vi "RTS MX4 Data.vi"(4 "Measurement Values in":dbl[][](array[numeric]), 6 "Debug":bool, 8 "Error In":errorcluster, 9 "Measurement Date Times":T1(array[cluster]), 10 "Chamber 1 Data in in":T4 {"Room PID Settings"."Room Dehumid Temperature I (*RM Dehum I1)" max=30000 step=1; "Room PID Settings"."Room Dehumid Temperature P (*RM Dehum P1)" max=30000 step=1; "Room PID Settings"."Room Cool Temperature I (*RM Cool I1)" max=30000 step=1; "Room PID Settings"."Room Cool Temperature P (*RM Cool P1)" max=30000 step=1; "Room PID Settings"."Room Heat I (*RM Heat I1)" max=30000 step=1; "Room PID Settings"."Room Heat P (*RM Heat P1)" max=30000 step=1; "Room PID Settings"."Room Humidity I (*RM Hum I1)" max=30000 step=1; "Room PID Settings"."Room Humidity P (*RM Hum P1)" max=30000 step=1; "Room PID Settings"."Room Dry I (*RM Dry I1)" max=30000 step=1; "Room PID Settings"."Room Dry P(*RM Dry P1)" max=30000 step=1; "Station 8"."Voltage (V):Element 1 Avg" format="%.3g"; "Station 8"."Voltage (V):Element 2 Avg" format="%.3g"; "Station 8"."Max Watt Hours" format="%.3g"; "Station 8"."Power Factor:Element 2" format="%.3g"; "Station 8"."Power Factor:Element 1" format="%.3g"; "Station 8"."Apparent Power (VA):Element 2" format="%.3g"; "Station 8"."Apparent Power (VA):Element 1" format="%.3g"; "Station 8"."Frequency (Hz):Element 1" format="%.3g"; "Station 8"."Time:Element 1" format="%.3g"; "Station 8"."Voltage Crest Factor:Element 2" format="%.3g"; "Station 8"."Voltage Crest Factor:Element 1" format="%.3g"; "Station 8"."Voltage Harmonic (%):Element 2" format="%.3g"; "Station 8"."Voltage Harmonic (%):Element 1" format="%.3g"; "Station 8"."Current Crest Factor:Element 2" format="%.3g"; "Station 8"."Current Crest Factor:Element 1" format="%.3g"; "Station 8"."Voltage (V):Element 1" format="%.3g"; "Station 8"."Voltage (V):Element 2" format="%.3g"; "Station 8"."Watt Hours (Wh):Sigma" format="%.3f"; "Station 8"."Power (W):Sigma" format="%.3g"; "Station 8"."Current (A):Element 2" format="%.3g"; "Station 8"."Current (A):Element 1" format="%.3g"; "Station 7"."Voltage (V):Element 1 Avg" format="%.3g"; "Station 7"."Voltage (V):Element 2 Avg" format="%.3g"; "Station 7"."Max Watt Hours" format="%.3g"; "Station 7"."Power Factor:Element 2" format="%.3g"; "Station 7"."Power Factor:Element 1" format="%.3g"; "Station 7"."Apparent Power (VA):Element 2" format="%.3g"; "Station 7"."Apparent Power (VA):Element 1" format="%.3g"; "Station 7"."Frequency (Hz):Element 1" format="%.3g"; "Station 7"."Time:Element 1" format="%.3g"; "Station 7"."Voltage Crest Factor:Element 2" format="%.3g"; "Station 7"."Voltage Crest Factor:Element 1" format="%.3g"; "Station 7"."Voltage Harmonic (%):Element 2" format="%.3g"; "Station 7"."Voltage Harmonic (%):Element 1" format="%.3g"; "Station 7"."Current Crest Factor:Element 2" format="%.3g"; "Station 7"."Current Crest Factor:Element 1" format="%.3g"; "Station 7"."Voltage (V):Element 1" format="%.3g"; "Station 7"."Voltage (V):Element 2" format="%.3g"; "Station 7"."Watt Hours (Wh):Sigma" format="%.3f"; "Station 7"."Power (W):Sigma" format="%.3g"; "Station 7"."Current (A):Element 2" format="%.3g"; "Station 7"."Current (A):Element 1" format="%.3g"; "Station 6"."Voltage (V):Element 1 Avg" format="%.3g"; "Station 6"."Voltage (V):Element 2 Avg" format="%.3g"; "Station 6"."Max Watt Hours" format="%.3g"; "Station 6"."Power Factor:Element 2" format="%.3g"; "Station 6"."Power Factor:Element 1" format="%.3g"; "Station 6"."Apparent Power (VA):Element 2" format="%.3g"; "Station 6"."Apparent Power (VA):Element 1" format="%.3g"; "Station 6"."Frequency (Hz):Element 1" format="%.3g"; "Station 6"."Time:Element 1" format="%.3g"; "Station 6"."Voltage Crest Factor:Element 2" format="%.3g"; "Station 6"."Voltage Crest Factor:Element 1" format="%.3g"; "Station 6"."Voltage Harmonic (%):Element 2" format="%.3g"; "Station 6"."Voltage Harmonic (%):Element 1" format="%.3g"; "Station 6"."Current Crest Factor:Element 2" format="%.3g"; "Station 6"."Current Crest Factor:Element 1" format="%.3g"; "Station 6"."Voltage (V):Element 1" format="%.3g"; "Station 6"."Voltage (V):Element 2" format="%.3g"; "Station 6"."Watt Hours (Wh):Sigma" format="%.3f"; "Station 6"."Power (W):Sigma" format="%.3g"; "Station 6"."Current (A):Element 2" format="%.3g"; "Station 6"."Current (A):Element 1" format="%.3g"; "Station 5"."Voltage (V):Element 1 Avg" format="%.3g"; "Station 5"."Voltage (V):Element 2 Avg" format="%.3g"; "Station 5"."Max Watt Hours" format="%.3g"; "Station 5"."Power Factor:Element 2" format="%.3g"; "Station 5"."Power Factor:Element 1" format="%.3g"; "Station 5"."Apparent Power (VA):Element 2" format="%.3g"; "Station 5"."Apparent Power (VA):Element 1" format="%.3g"; "Station 5"."Frequency (Hz):Element 1" format="%.3g"; "Station 5"."Time:Element 1" format="%.3g"; "Station 5"."Voltage Crest Factor:Element 2" format="%.3g"; "Station 5"."Voltage Crest Factor:Element 1" format="%.3g"; "Station 5"."Voltage Harmonic (%):Element 2" format="%.3g"; "Station 5"."Voltage Harmonic (%):Element 1" format="%.3g"; "Station 5"."Current Crest Factor:Element 2" format="%.3g"; "Station 5"."Current Crest Factor:Element 1" format="%.3g"; "Station 5"."Voltage (V):Element 1" format="%.3g"; "Station 5"."Voltage (V):Element 2" format="%.3g"; "Station 5"."Watt Hours (Wh):Sigma" format="%.3f"; "Station 5"."Power (W):Sigma" format="%.3g"; "Station 5"."Current (A):Element 2" format="%.3g"; "Station 5"."Current (A):Element 1" format="%.3g"; "Station 4"."Voltage (V):Element 1 Avg" format="%.3g"; "Station 4"."Voltage (V):Element 2 Avg" format="%.3g"; "Station 4"."Max Watt Hours" format="%.3g"; "Station 4"."Power Factor:Element 2" format="%.3g"; "Station 4"."Power Factor:Element 1" format="%.3g"; "Station 4"."Apparent Power (VA):Element 2" format="%.3g"; "Station 4"."Apparent Power (VA):Element 1" format="%.3g"; "Station 4"."Frequency (Hz):Element 1" format="%.3g"; "Station 4"."Time:Element 1" format="%.3g"; "Station 4"."Voltage Crest Factor:Element 2" format="%.3g"; "Station 4"."Voltage Crest Factor:Element 1" format="%.3g"; "Station 4"."Voltage Harmonic (%):Element 2" format="%.3g"; "Station 4"."Voltage Harmonic (%):Element 1" format="%.3g"; "Station 4"."Current Crest Factor:Element 2" format="%.3g"; "Station 4"."Current Crest Factor:Element 1" format="%.3g"; "Station 4"."Voltage (V):Element 1" format="%.3g"; "Station 4"."Voltage (V):Element 2" format="%.3g"; "Station 4"."Watt Hours (Wh):Sigma" format="%.3f"; "Station 4"."Power (W):Sigma" format="%.3g"; "Station 4"."Current (A):Element 2" format="%.3g"; "Station 4"."Current (A):Element 1" format="%.3g"; "Station 3"."Voltage (V):Element 1 Avg" format="%.3g"; "Station 3"."Voltage (V):Element 2 Avg" format="%.3g"; "Station 3"."Max Watt Hours" format="%.3g"; "Station 3"."Power Factor:Element 2" format="%.3g"; "Station 3"."Power Factor:Element 1" format="%.3g"; "Station 3"."Apparent Power (VA):Element 2" format="%.3g"; "Station 3"."Apparent Power (VA):Element 1" format="%.3g"; "Station 3"."Frequency (Hz):Element 1" format="%.3g"; "Station 3"."Time:Element 1" format="%.3g"; "Station 3"."Voltage Crest Factor:Element 2" format="%.3g"; "Station 3"."Voltage Crest Factor:Element 1" format="%.3g"; "Station 3"."Voltage Harmonic (%):Element 2" format="%.3g"; "Station 3"."Voltage Harmonic (%):Element 1" format="%.3g"; "Station 3"."Current Crest Factor:Element 2" format="%.3g"; "Station 3"."Current Crest Factor:Element 1" format="%.3g"; "Station 3"."Voltage (V):Element 1" format="%.3g"; "Station 3"."Voltage (V):Element 2" format="%.3g"; "Station 3"."Watt Hours (Wh):Sigma" format="%.3f"; "Station 3"."Power (W):Sigma" format="%.3g"; "Station 3"."Current (A):Element 2" format="%.3g"; "Station 3"."Current (A):Element 1" format="%.3g"; "Station 2"."Voltage (V):Element 1 Avg" format="%.3g"; "Station 2"."Voltage (V):Element 2 Avg" format="%.3g"; "Station 2"."Max Watt Hours" format="%.3g"; "Station 2"."Power Factor:Element 2" format="%.3g"; "Station 2"."Power Factor:Element 1" format="%.3g"; "Station 2"."Apparent Power (VA):Element 2" format="%.3g"; "Station 2"."Apparent Power (VA):Element 1" format="%.3g"; "Station 2"."Frequency (Hz):Element 1" format="%.3g"; "Station 2"."Time:Element 1" format="%.3g"; "Station 2"."Voltage Crest Factor:Element 2" format="%.3g"; "Station 2"."Voltage Crest Factor:Element 1" format="%.3g"; "Station 2"."Voltage Harmonic (%):Element 2" format="%.3g"; "Station 2"."Voltage Harmonic (%):Element 1" format="%.3g"; "Station 2"."Current Crest Factor:Element 2" format="%.3g"; "Station 2"."Current Crest Factor:Element 1" format="%.3g"; "Station 2"."Voltage (V):Element 1" format="%.3g"; "Station 2"."Voltage (V):Element 2" format="%.3g"; "Station 2"."Watt Hours (Wh):Sigma" format="%.3f"; "Station 2"."Power (W):Sigma" format="%.3g"; "Station 2"."Current (A):Element 2" format="%.3g"; "Station 2"."Current (A):Element 1" format="%.3g"; "Station 1"."Voltage (V):Element 1 Avg" format="%.3g"; "Station 1"."Voltage (V):Element 2 Avg" format="%.3g"; "Station 1"."Max Watt Hours" format="%.3g"; "Station 1"."Power Factor:Element 2" format="%.3g"; "Station 1"."Power Factor:Element 1" format="%.3g"; "Station 1"."Apparent Power (VA):Element 2" format="%.3g"; "Station 1"."Apparent Power (VA):Element 1" format="%.3g"; "Station 1"."Frequency (Hz):Element 1" format="%.3g"; "Station 1"."Time:Element 1" format="%.3g"; "Station 1"."Voltage Crest Factor:Element 2" format="%.3g"; "Station 1"."Voltage Crest Factor:Element 1" format="%.3g"; "Station 1"."Voltage Harmonic (%):Element 2" format="%.3g"; "Station 1"."Voltage Harmonic (%):Element 1" format="%.3g"; "Station 1"."Current Crest Factor:Element 2" format="%.3g"; "Station 1"."Current Crest Factor:Element 1" format="%.3g"; "Station 1"."Voltage (V):Element 1" format="%.3g"; "Station 1"."Voltage (V):Element 2" format="%.3g"; "Station 1"."Watt Hours (Wh):Sigma" format="%.3f"; "Station 1"."Power (W):Sigma" format="%.3g"; "Station 1"."Current (A):Element 2" format="%.3g"; "Station 1"."Current (A):Element 1" format="%.3g"}, 11 "MX":T2={"Base Time"=0, "Session Number"=0, "Last Data Number"={"High"=-1, "Low"=4294967295}, "Channel List"=[], "FIFO Number (0)"=0, "Channel Number (1)"=1, "Select FIFO or Channel (F:Channel)"=FALSE, "MX100 Data"={"Measurement Values out"=[], "Date/Time"=""}} {"Channel Number (1)" min=1 max=60 step=1; "FIFO Number (0)" min=-1 max=2 step=1}) -> (0 "Error Out":errorcluster, 2 "Chamber 1 Data out":T4 {"Room PID Settings"."Room Dehumid Temperature I (*RM Dehum I1)" max=30000 step=1; "Room PID Settings"."Room Dehumid Temperature P (*RM Dehum P1)" max=30000 step=1; "Room PID Settings"."Room Cool Temperature I (*RM Cool I1)" max=30000 step=1; "Room PID Settings"."Room Cool Temperature P (*RM Cool P1)" max=30000 step=1; "Room PID Settings"."Room Heat I (*RM Heat I1)" max=30000 step=1; "Room PID Settings"."Room Heat P (*RM Heat P1)" max=30000 step=1; "Room PID Settings"."Room Humidity I (*RM Hum I1)" max=30000 step=1; "Room PID Settings"."Room Humidity P (*RM Hum P1)" max=30000 step=1; "Room PID Settings"."Room Dry I (*RM Dry I1)" max=30000 step=1; "Room PID Settings"."Room Dry P(*RM Dry P1)" max=30000 step=1; "Station 8"."Voltage (V):Element 1 Avg" format="%.3g"; "Station 8"."Voltage (V):Element 2 Avg" format="%.3g"; "Station 8"."Max Watt Hours" format="%.3g"; "Station 8"."Power Factor:Element 2" format="%.3g"; "Station 8"."Power Factor:Element 1" format="%.3g"; "Station 8"."Apparent Power (VA):Element 2" format="%.3g"; "Station 8"."Apparent Power (VA):Element 1" format="%.3g"; "Station 8"."Frequency (Hz):Element 1" format="%.3g"; "Station 8"."Time:Element 1" format="%.3g"; "Station 8"."Voltage Crest Factor:Element 2" format="%.3g"; "Station 8"."Voltage Crest Factor:Element 1" format="%.3g"; "Station 8"."Voltage Harmonic (%):Element 2" format="%.3g"; "Station 8"."Voltage Harmonic (%):Element 1" format="%.3g"; "Station 8"."Current Crest Factor:Element 2" format="%.3g"; "Station 8"."Current Crest Factor:Element 1" format="%.3g"; "Station 8"."Voltage (V):Element 1" format="%.3g"; "Station 8"."Voltage (V):Element 2" format="%.3g"; "Station 8"."Watt Hours (Wh):Sigma" format="%.3f"; "Station 8"."Power (W):Sigma" format="%.3g"; "Station 8"."Current (A):Element 2" format="%.3g"; "Station 8"."Current (A):Element 1" format="%.3g"; "Station 7"."Voltage (V):Element 1 Avg" format="%.3g"; "Station 7"."Voltage (V):Element 2 Avg" format="%.3g"; "Station 7"."Max Watt Hours" format="%.3g"; "Station 7"."Power Factor:Element 2" format="%.3g"; "Station 7"."Power Factor:Element 1" format="%.3g"; "Station 7"."Apparent Power (VA):Element 2" format="%.3g"; "Station 7"."Apparent Power (VA):Element 1" format="%.3g"; "Station 7"."Frequency (Hz):Element 1" format="%.3g"; "Station 7"."Time:Element 1" format="%.3g"; "Station 7"."Voltage Crest Factor:Element 2" format="%.3g"; "Station 7"."Voltage Crest Factor:Element 1" format="%.3g"; "Station 7"."Voltage Harmonic (%):Element 2" format="%.3g"; "Station 7"."Voltage Harmonic (%):Element 1" format="%.3g"; "Station 7"."Current Crest Factor:Element 2" format="%.3g"; "Station 7"."Current Crest Factor:Element 1" format="%.3g"; "Station 7"."Voltage (V):Element 1" format="%.3g"; "Station 7"."Voltage (V):Element 2" format="%.3g"; "Station 7"."Watt Hours (Wh):Sigma" format="%.3f"; "Station 7"."Power (W):Sigma" format="%.3g"; "Station 7"."Current (A):Element 2" format="%.3g"; "Station 7"."Current (A):Element 1" format="%.3g"; "Station 6"."Voltage (V):Element 1 Avg" format="%.3g"; "Station 6"."Voltage (V):Element 2 Avg" format="%.3g"; "Station 6"."Max Watt Hours" format="%.3g"; "Station 6"."Power Factor:Element 2" format="%.3g"; "Station 6"."Power Factor:Element 1" format="%.3g"; "Station 6"."Apparent Power (VA):Element 2" format="%.3g"; "Station 6"."Apparent Power (VA):Element 1" format="%.3g"; "Station 6"."Frequency (Hz):Element 1" format="%.3g"; "Station 6"."Time:Element 1" format="%.3g"; "Station 6"."Voltage Crest Factor:Element 2" format="%.3g"; "Station 6"."Voltage Crest Factor:Element 1" format="%.3g"; "Station 6"."Voltage Harmonic (%):Element 2" format="%.3g"; "Station 6"."Voltage Harmonic (%):Element 1" format="%.3g"; "Station 6"."Current Crest Factor:Element 2" format="%.3g"; "Station 6"."Current Crest Factor:Element 1" format="%.3g"; "Station 6"."Voltage (V):Element 1" format="%.3g"; "Station 6"."Voltage (V):Element 2" format="%.3g"; "Station 6"."Watt Hours (Wh):Sigma" format="%.3f"; "Station 6"."Power (W):Sigma" format="%.3g"; "Station 6"."Current (A):Element 2" format="%.3g"; "Station 6"."Current (A):Element 1" format="%.3g"; "Station 5"."Voltage (V):Element 1 Avg" format="%.3g"; "Station 5"."Voltage (V):Element 2 Avg" format="%.3g"; "Station 5"."Max Watt Hours" format="%.3g"; "Station 5"."Power Factor:Element 2" format="%.3g"; "Station 5"."Power Factor:Element 1" format="%.3g"; "Station 5"."Apparent Power (VA):Element 2" format="%.3g"; "Station 5"."Apparent Power (VA):Element 1" format="%.3g"; "Station 5"."Frequency (Hz):Element 1" format="%.3g"; "Station 5"."Time:Element 1" format="%.3g"; "Station 5"."Voltage Crest Factor:Element 2" format="%.3g"; "Station 5"."Voltage Crest Factor:Element 1" format="%.3g"; "Station 5"."Voltage Harmonic (%):Element 2" format="%.3g"; "Station 5"."Voltage Harmonic (%):Element 1" format="%.3g"; "Station 5"."Current Crest Factor:Element 2" format="%.3g"; "Station 5"."Current Crest Factor:Element 1" format="%.3g"; "Station 5"."Voltage (V):Element 1" format="%.3g"; "Station 5"."Voltage (V):Element 2" format="%.3g"; "Station 5"."Watt Hours (Wh):Sigma" format="%.3f"; "Station 5"."Power (W):Sigma" format="%.3g"; "Station 5"."Current (A):Element 2" format="%.3g"; "Station 5"."Current (A):Element 1" format="%.3g"; "Station 4"."Voltage (V):Element 1 Avg" format="%.3g"; "Station 4"."Voltage (V):Element 2 Avg" format="%.3g"; "Station 4"."Max Watt Hours" format="%.3g"; "Station 4"."Power Factor:Element 2" format="%.3g"; "Station 4"."Power Factor:Element 1" format="%.3g"; "Station 4"."Apparent Power (VA):Element 2" format="%.3g"; "Station 4"."Apparent Power (VA):Element 1" format="%.3g"; "Station 4"."Frequency (Hz):Element 1" format="%.3g"; "Station 4"."Time:Element 1" format="%.3g"; "Station 4"."Voltage Crest Factor:Element 2" format="%.3g"; "Station 4"."Voltage Crest Factor:Element 1" format="%.3g"; "Station 4"."Voltage Harmonic (%):Element 2" format="%.3g"; "Station 4"."Voltage Harmonic (%):Element 1" format="%.3g"; "Station 4"."Current Crest Factor:Element 2" format="%.3g"; "Station 4"."Current Crest Factor:Element 1" format="%.3g"; "Station 4"."Voltage (V):Element 1" format="%.3g"; "Station 4"."Voltage (V):Element 2" format="%.3g"; "Station 4"."Watt Hours (Wh):Sigma" format="%.3f"; "Station 4"."Power (W):Sigma" format="%.3g"; "Station 4"."Current (A):Element 2" format="%.3g"; "Station 4"."Current (A):Element 1" format="%.3g"; "Station 3"."Voltage (V):Element 1 Avg" format="%.3g"; "Station 3"."Voltage (V):Element 2 Avg" format="%.3g"; "Station 3"."Max Watt Hours" format="%.3g"; "Station 3"."Power Factor:Element 2" format="%.3g"; "Station 3"."Power Factor:Element 1" format="%.3g"; "Station 3"."Apparent Power (VA):Element 2" format="%.3g"; "Station 3"."Apparent Power (VA):Element 1" format="%.3g"; "Station 3"."Frequency (Hz):Element 1" format="%.3g"; "Station 3"."Time:Element 1" format="%.3g"; "Station 3"."Voltage Crest Factor:Element 2" format="%.3g"; "Station 3"."Voltage Crest Factor:Element 1" format="%.3g"; "Station 3"."Voltage Harmonic (%):Element 2" format="%.3g"; "Station 3"."Voltage Harmonic (%):Element 1" format="%.3g"; "Station 3"."Current Crest Factor:Element 2" format="%.3g"; "Station 3"."Current Crest Factor:Element 1" format="%.3g"; "Station 3"."Voltage (V):Element 1" format="%.3g"; "Station 3"."Voltage (V):Element 2" format="%.3g"; "Station 3"."Watt Hours (Wh):Sigma" format="%.3f"; "Station 3"."Power (W):Sigma" format="%.3g"; "Station 3"."Current (A):Element 2" format="%.3g"; "Station 3"."Current (A):Element 1" format="%.3g"; "Station 2"."Voltage (V):Element 1 Avg" format="%.3g"; "Station 2"."Voltage (V):Element 2 Avg" format="%.3g"; "Station 2"."Max Watt Hours" format="%.3g"; "Station 2"."Power Factor:Element 2" format="%.3g"; "Station 2"."Power Factor:Element 1" format="%.3g"; "Station 2"."Apparent Power (VA):Element 2" format="%.3g"; "Station 2"."Apparent Power (VA):Element 1" format="%.3g"; "Station 2"."Frequency (Hz):Element 1" format="%.3g"; "Station 2"."Time:Element 1" format="%.3g"; "Station 2"."Voltage Crest Factor:Element 2" format="%.3g"; "Station 2"."Voltage Crest Factor:Element 1" format="%.3g"; "Station 2"."Voltage Harmonic (%):Element 2" format="%.3g"; "Station 2"."Voltage Harmonic (%):Element 1" format="%.3g"; "Station 2"."Current Crest Factor:Element 2" format="%.3g"; "Station 2"."Current Crest Factor:Element 1" format="%.3g"; "Station 2"."Voltage (V):Element 1" format="%.3g"; "Station 2"."Voltage (V):Element 2" format="%.3g"; "Station 2"."Watt Hours (Wh):Sigma" format="%.3f"; "Station 2"."Power (W):Sigma" format="%.3g"; "Station 2"."Current (A):Element 2" format="%.3g"; "Station 2"."Current (A):Element 1" format="%.3g"; "Station 1"."Voltage (V):Element 1 Avg" format="%.3g"; "Station 1"."Voltage (V):Element 2 Avg" format="%.3g"; "Station 1"."Max Watt Hours" format="%.3g"; "Station 1"."Power Factor:Element 2" format="%.3g"; "Station 1"."Power Factor:Element 1" format="%.3g"; "Station 1"."Apparent Power (VA):Element 2" format="%.3g"; "Station 1"."Apparent Power (VA):Element 1" format="%.3g"; "Station 1"."Frequency (Hz):Element 1" format="%.3g"; "Station 1"."Time:Element 1" format="%.3g"; "Station 1"."Voltage Crest Factor:Element 2" format="%.3g"; "Station 1"."Voltage Crest Factor:Element 1" format="%.3g"; "Station 1"."Voltage Harmonic (%):Element 2" format="%.3g"; "Station 1"."Voltage Harmonic (%):Element 1" format="%.3g"; "Station 1"."Current Crest Factor:Element 2" format="%.3g"; "Station 1"."Current Crest Factor:Element 1" format="%.3g"; "Station 1"."Voltage (V):Element 1" format="%.3g"; "Station 1"."Voltage (V):Element 2" format="%.3g"; "Station 1"."Watt Hours (Wh):Sigma" format="%.3f"; "Station 1"."Power (W):Sigma" format="%.3g"; "Station 1"."Current (A):Element 2" format="%.3g"; "Station 1"."Current (A):Element 1" format="%.3g"})   [LabVIEW 2016]
uses:
  Type Definitions/RTS Chamber Data.ctl
  Utility/Type Definitions/UTILITY Power Data.ctl
  Type Definitions/RTS Chamber TCs.ctl
  Type Definitions/RTS MX5 AUX Data.ctl
  Drivers/WAGO 750-881/Type Definitions/Wago Door Relays.ctl
  Drivers/WAGO 750-881/Type Definitions/Wago Contactor Settings.ctl
  Drivers/WAGO 750-881/Type Definitions/Wago Ground Leakage.ctl
  Drivers/WAGO 750-881/Type Definitions/Wago Measured Input Data.ctl
  Drivers/WAGO 750-881/Type Definitions/Wago Room Setpoint Targets.ctl
  Drivers/WAGO 750-881/Type Definitions/Wago Room PID Settings.ctl
  Drivers/WAGO 750-881/Type Definitions/Wago Room Condtions.ctl
  Drivers/Yokogawa MX100/Type Definitions/MX100 Initialization.ctl
  Drivers/Yokogawa MX100/Type Definitions/MX100 Data.ctl
panel:
  # "APLUS"
  # "MX100"
  # "Wago Controller"
  # "APLUS"
  # "MX100"
  # "Wago Controller"
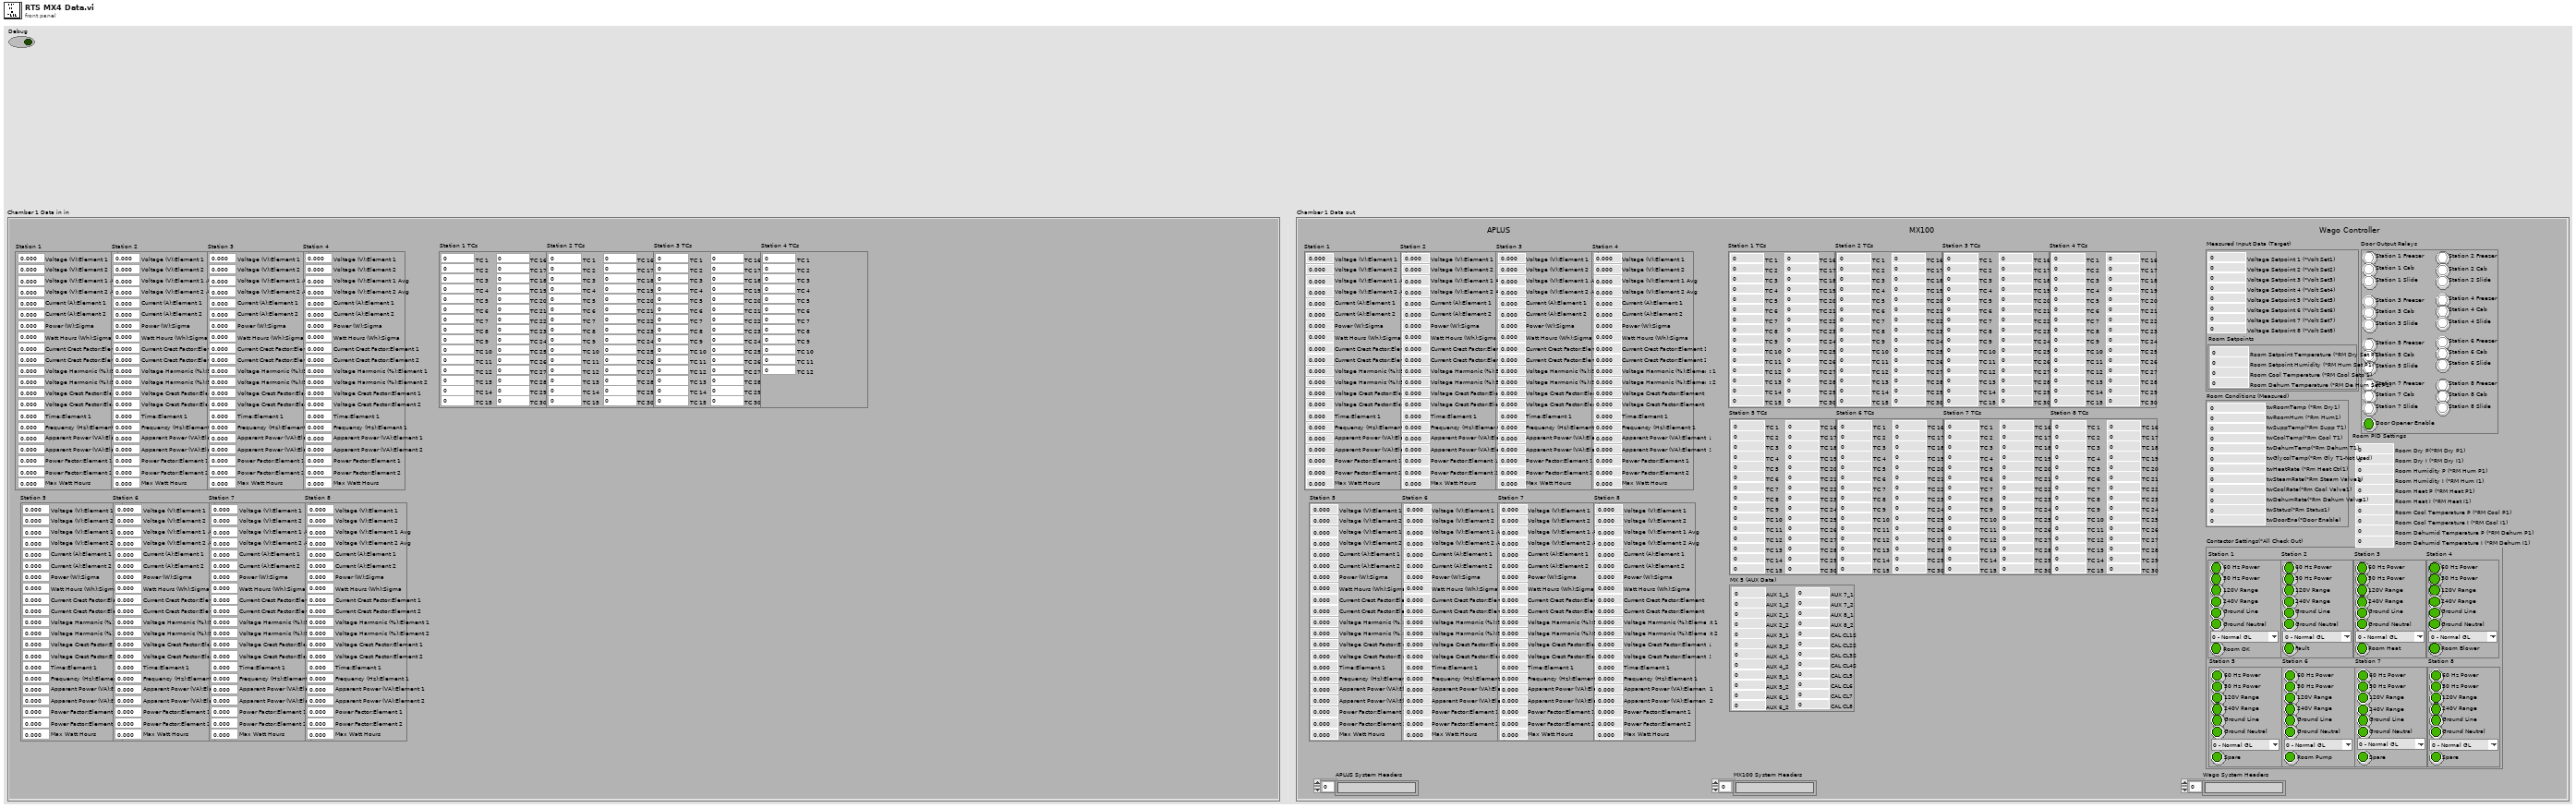
[diagram p1: front panel]
types:
  T1 = cluster{"Measurement Time":u32, "Milli Second":i32}[]
  T2 = typedef "MX100 Initialization.ctl" = cluster{"Base Time":i32, "Session Number":i32, "Last Data Number":cluster{"High":i32, "Low":u32}, "Channel List":string[], "FIFO Number (0)":i32, "Channel Number (1)":i32, "Select FIFO or Channel (F:Channel)":bool, "MX100 Data":T3}
  T3 = typedef "MX100 Data.ctl" = cluster{"Measurement Values out":dbl[], "Date/Time":string}
  T4 = typedef "RTS Chamber Data.ctl" = cluster{"Station 1":T5, "Station 2":T5, "Station 3":T5, "Station 4":T5, "Station 5":T5, "Station 6":T5, "Station 7":T5, "Station 8":T5, "Station 1 TCs":T6, "Station 2 TCs":T6, "Station 3 TCs":T6, "Station 4 TCs":T6, "Station 5 TCs":T6, "Station 6 TCs":T6, "Station 7 TCs":T6, "Station 8 TCs":T6, "MX 5 (AUX Data)":T7, "Door Output Relays":T8, "Contactor Settings(*All Check Out)":T9, "Measured Input Data (Target)":T11, "Room PID Settings":T13, "Room Conditions (Measured)":T14, "APLUS System Headers":string[], "MX100 System Headers":string[], "Wago System Headers":string[]}
  T5 = typedef "UTILITY Power Data.ctl" = cluster{"Current (A):Element 1":dbl, "Current (A):Element 2":dbl, "Power (W):Sigma":dbl, "Watt Hours (Wh):Sigma":dbl, "Voltage (V):Element 2":dbl, "Voltage (V):Element 1":dbl, "Current Crest Factor:Element 1":dbl, "Current Crest Factor:Element 2":dbl, "Voltage Harmonic (%):Element 1":dbl, "Voltage Harmonic (%):Element 2":dbl, "Voltage Crest Factor:Element 1":dbl, "Voltage Crest Factor:Element 2":dbl, "Time:Element 1":dbl, "Frequency (Hz):Element 1":dbl, "Apparent Power (VA):Element 1":dbl, "Apparent Power (VA):Element 2":dbl, "Power Factor:Element 1":dbl, "Power Factor:Element 2":dbl, "Max Watt Hours":dbl, "Voltage (V):Element 2 Avg":dbl, "Voltage (V):Element 1 Avg":dbl}
  T6 = typedef "RTS Chamber TCs.ctl" = cluster{"TC 1":dbl, "TC 2":dbl, "TC 3":dbl, "TC 4":dbl, "TC 5":dbl, "TC 6":dbl, "TC 7":dbl, "TC 8":dbl, "TC 9":dbl, "TC 10":dbl, "TC 11":dbl, "TC 12":dbl, "TC 13":dbl, "TC 14":dbl, "TC 15":dbl, "TC 16":dbl, "TC 17":dbl, "TC 18":dbl, "TC 19":dbl, "TC 20":dbl, "TC 21":dbl, "TC 22":dbl, "TC 23":dbl, "TC 24":dbl, "TC 25":dbl, "TC 26":dbl, "TC 27":dbl, "TC 28":dbl, "TC 29":dbl, "TC 30":dbl}
  T7 = typedef "RTS MX5 AUX Data.ctl" = cluster{"AUX 1_1":dbl, "AUX 1_2":dbl, "AUX 2_1":dbl, "AUX 2_2":dbl, "AUX 3_1":dbl, "AUX 3_2":dbl, "AUX 4_1":dbl, "AUX 4_2":dbl, "AUX 5_1":dbl, "AUX 5_2":dbl, "AUX 6_1":dbl, "AUX 6_2":dbl, "AUX 7_1":dbl, "AUX 7_2":dbl, "AUX 8_1":dbl, "AUX 8_2":dbl, "CAL CL1S":dbl, "CAL CL2S":dbl, "CAL CL3S":dbl, "CAL CL4S":dbl, "CAL CL5":dbl, "CAL CL6":dbl, "CAL CL7":dbl, "CAL CL8":dbl}
  T8 = typedef "Wago Door Relays.ctl" = cluster{"Station 1 Freezer":bool, "Station 1 Cab":bool, "Station 1 Slide":bool, "Station 2 Freezer":bool, "Station 2 Cab":bool, "Station 2 Slide":bool, "Station 3 Freezer":bool, "Station 3 Cab":bool, "Station 3 Slide":bool, "Station 4 Freezer":bool, "Station 4 Cab":bool, "Station 4 Slide":bool, "Station 5 Freezer":bool, "Station 5 Cab":bool, "Station 5 Slide":bool, "Station 6 Freezer":bool, "Station 6 Cab":bool, "Station 6 Slide":bool, "Station 7 Freezer":bool, "Station 7 Cab":bool, "Station 7 Slide":bool, "Station 8 Freezer":bool, "Station 8 Cab":bool, "Station 8 Slide":bool, "Door Opener Enable":bool}
  T9 = typedef "Wago Contactor Settings.ctl" = cluster{"Station 1":cluster{"60 Hz Power":bool, "50 Hz Power":bool, "120V Range":bool, "240V Range":bool, "Ground Line":bool, "Ground Neutral":bool, "Room OK":bool, "Ground Leakage":T10}, "Station 2":cluster{"60 Hz Power":bool, "50 Hz Power":bool, "120V Range":bool, "240V Range":bool, "Ground Line":bool, "Ground Neutral":bool, "Fault":bool, "Ground Leakage":T10}, "Station 3":cluster{"60 Hz Power":bool, "50 Hz Power":bool, "120V Range":bool, "240V Range":bool, "Ground Line":bool, "Ground Neutral":bool, "Room Heat":bool, "Ground Leakage":T10}, "Station 4":cluster{"60 Hz Power":bool, "50 Hz Power":bool, "120V Range":bool, "240V Range":bool, "Ground Line":bool, "Ground Neutral":bool, "Room Blower":bool, "Ground Leakage":T10}, "Station 5":cluster{"60 Hz Power":bool, "50 Hz Power":bool, "120V Range":bool, "240V Range":bool, "Ground Line":bool, "Ground Neutral":bool, "Spare":bool, "Ground Leakage":T10}, "Station 6":cluster{"60 Hz Power":bool, "50 Hz Power":bool, "120V Range":bool, "240V Range":bool, "Ground Line":bool, "Ground Neutral":bool, "Room Pump":bool, "Ground Leakage":T10}, "Station 7":cluster{"60 Hz Power":bool, "50 Hz Power":bool, "120V Range":bool, "240V Range":bool, "Ground Line":bool, "Ground Neutral":bool, "Spare":bool, "Ground Leakage":T10}, "Station 8":cluster{"60 Hz Power":bool, "50 Hz Power":bool, "120V Range":bool, "240V Range":bool, "Ground Line":bool, "Ground Neutral":bool, "Spare":bool, "Ground Leakage":T10}}
  T10 = typedef "Wago Ground Leakage.ctl" = enum16{"0 - Normal GL", "1 - Measure GL"}
  T11 = typedef "Wago Measured Input Data.ctl" = cluster{"Voltage Setpoint 1 (*Volt Set1)":dbl, "Voltage Setpoint 2 (*Volt Set2)":dbl, "Voltage Setpoint 3 (*Volt Set3)":dbl, "Voltage Setpoint 4 (*Volt Set4)":dbl, "Voltage Setpoint 5 (*Volt Set5)":dbl, "Voltage Setpoint 6 (*Volt Set6)":dbl, "Voltage Setpoint 7 (*Volt Set7)":dbl, "Voltage Setpoint 8 (*Volt Set8)":dbl, "Room Setpoints":T12}
  T12 = typedef "Wago Room Setpoint Targets.ctl" = cluster{"Room Setpoint Temperature (*RM Dry Set P1)":dbl, "Room Setpoint Humidity (*RM Hum Set P1)":dbl, "Room Cool Temperature (*RM Cool Setp 1)":dbl, "Room Dehum Temperature (*RM De Hum Set P1)":dbl}
  T13 = typedef "Wago Room PID Settings.ctl" = cluster{"Room Dry P(*RM Dry P1)":u16, "Room Dry I (*RM Dry I1)":u16, "Room Humidity P (*RM Hum P1)":u16, "Room Humidity I (*RM Hum I1)":u16, "Room Heat P (*RM Heat P1)":u16, "Room Heat I (*RM Heat I1)":u16, "Room Cool Temperature P (*RM Cool P1)":u16, "Room Cool Temperature I (*RM Cool I1)":u16, "Room Dehumid Temperature P (*RM Dehum P1)":u16, "Room Dehumid Temperature I (*RM Dehum I1)":u16}
  T14 = typedef "Wago Room Condtions.ctl" = cluster{"twDoorEna(*Door Enable)":u16, "twStatus(*Rm Status1)":u16, "twRoomTemp (*Rm Dry1)":dbl, "twRoomHum (*Rm Hum1)":dbl, "twSuppTemp(*Rm Supp T1)":dbl, "twCoolTemp(*Rm Cool T1)":dbl, "twDehumTemp(*Rm Dehum T1)":dbl, "twGlycolTemp(*Rm Gly T1-Not Used)":dbl, "twDehumRate(*Rm Dehum Valve1)":dbl, "twCoolRate(*Rm Cool Valve1)":dbl, "twSteamRate(*Rm Steam Valve1)":dbl, "twHeatRate (*Rm Heat Ctrl1)":dbl}
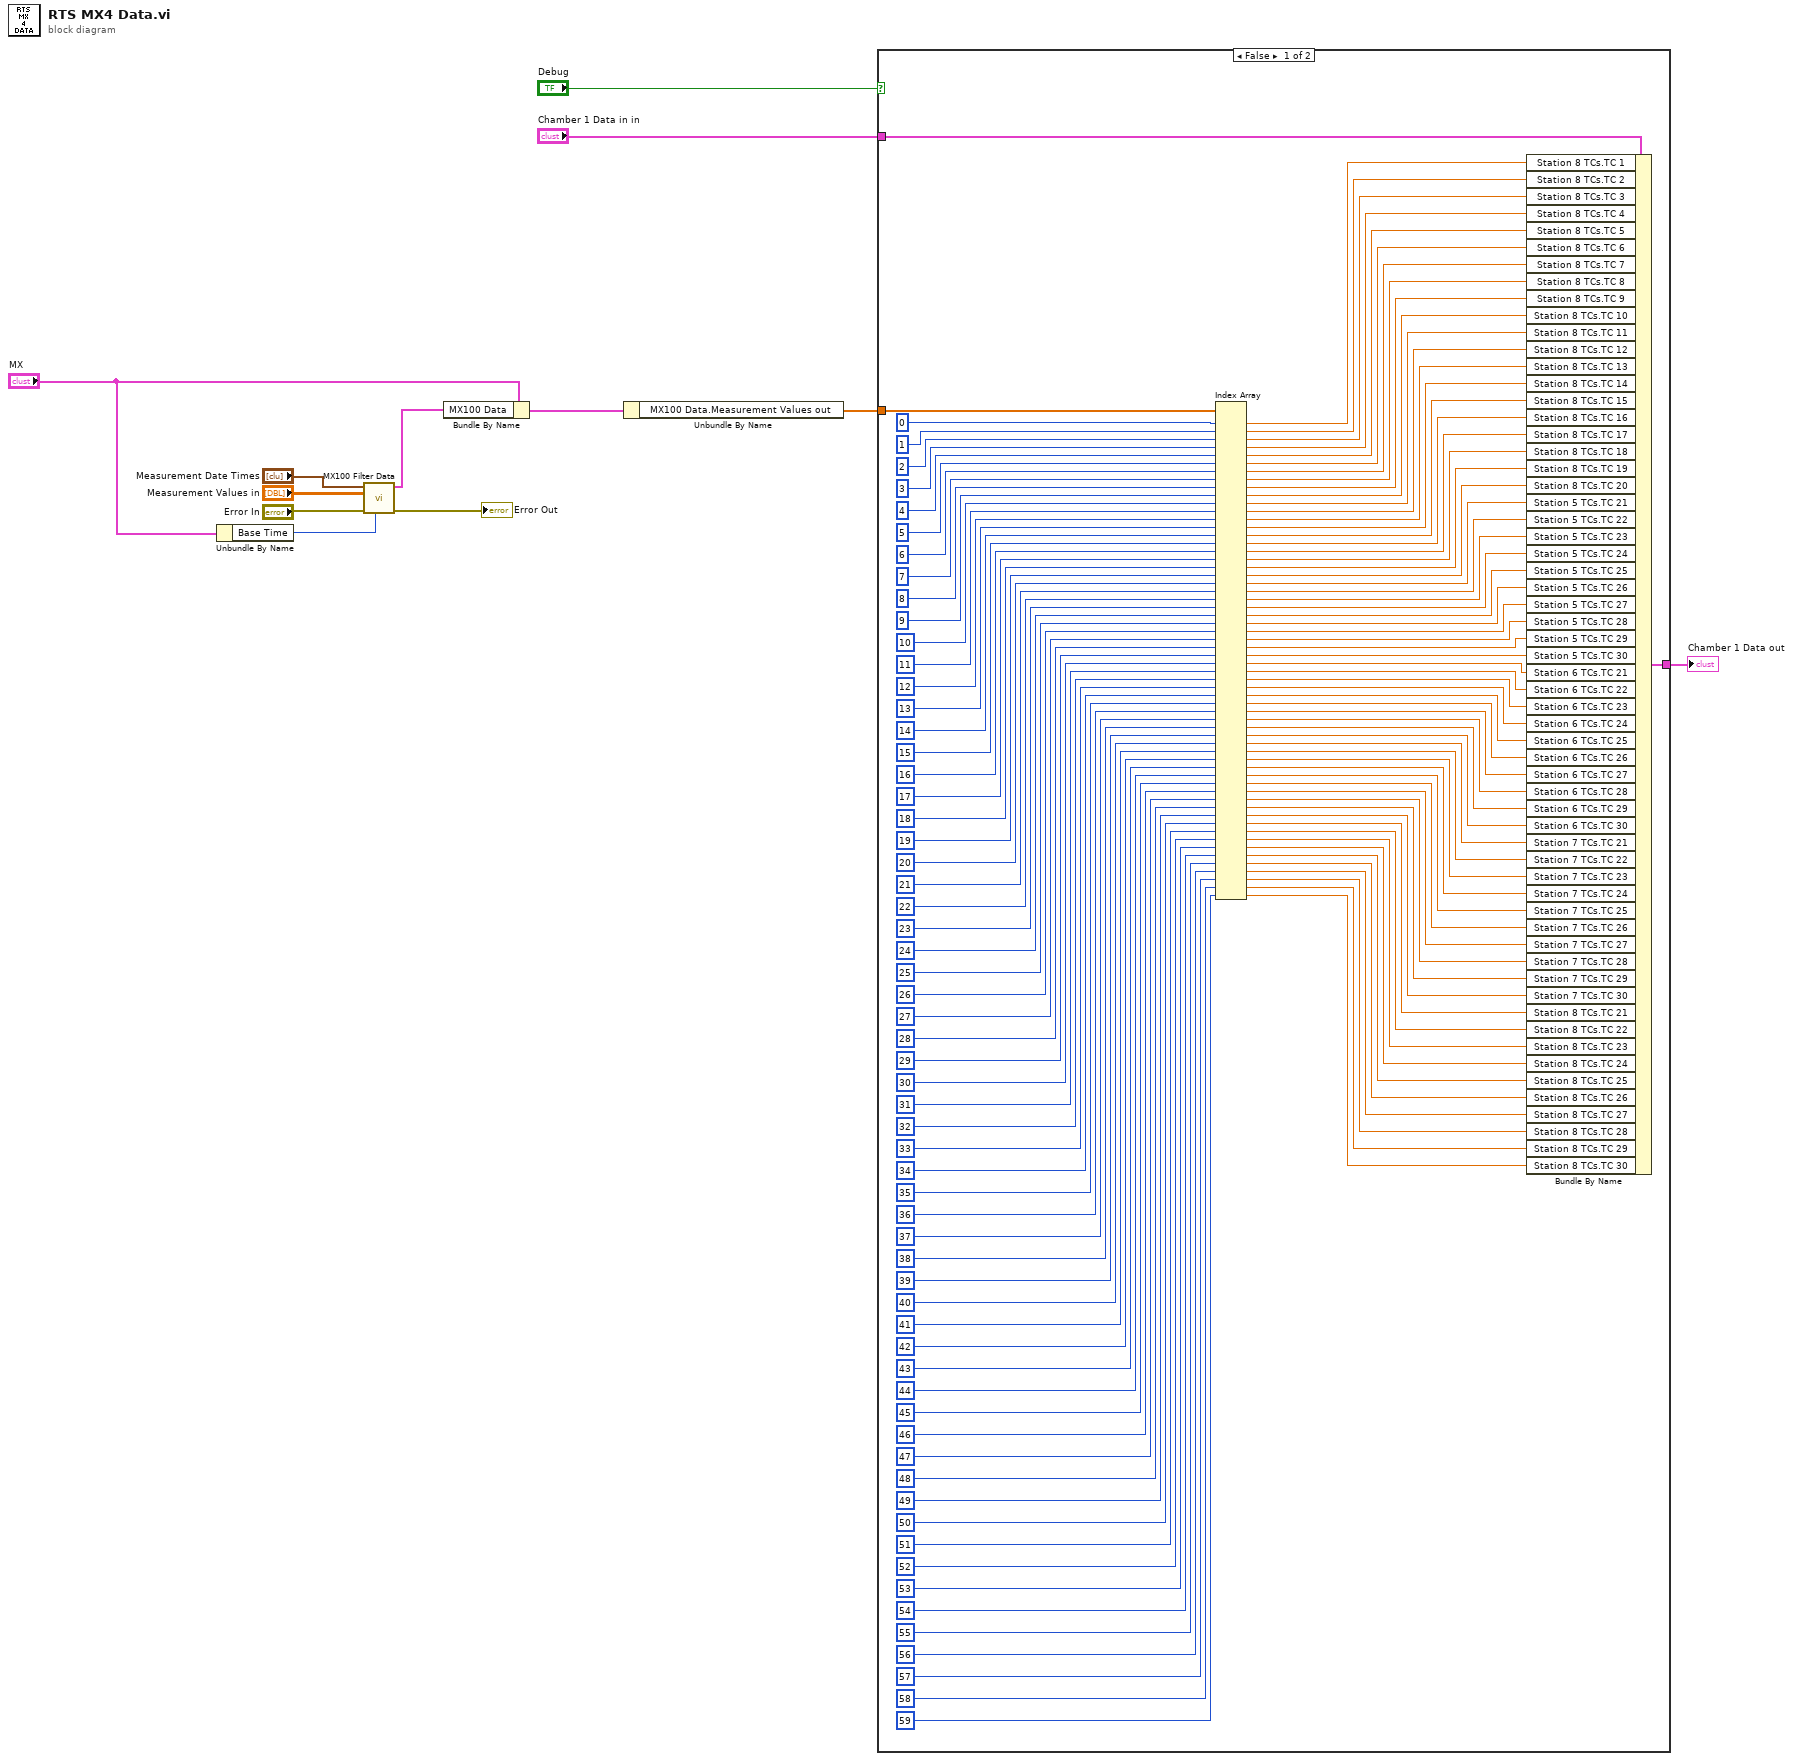
[diagram p0: block diagram]
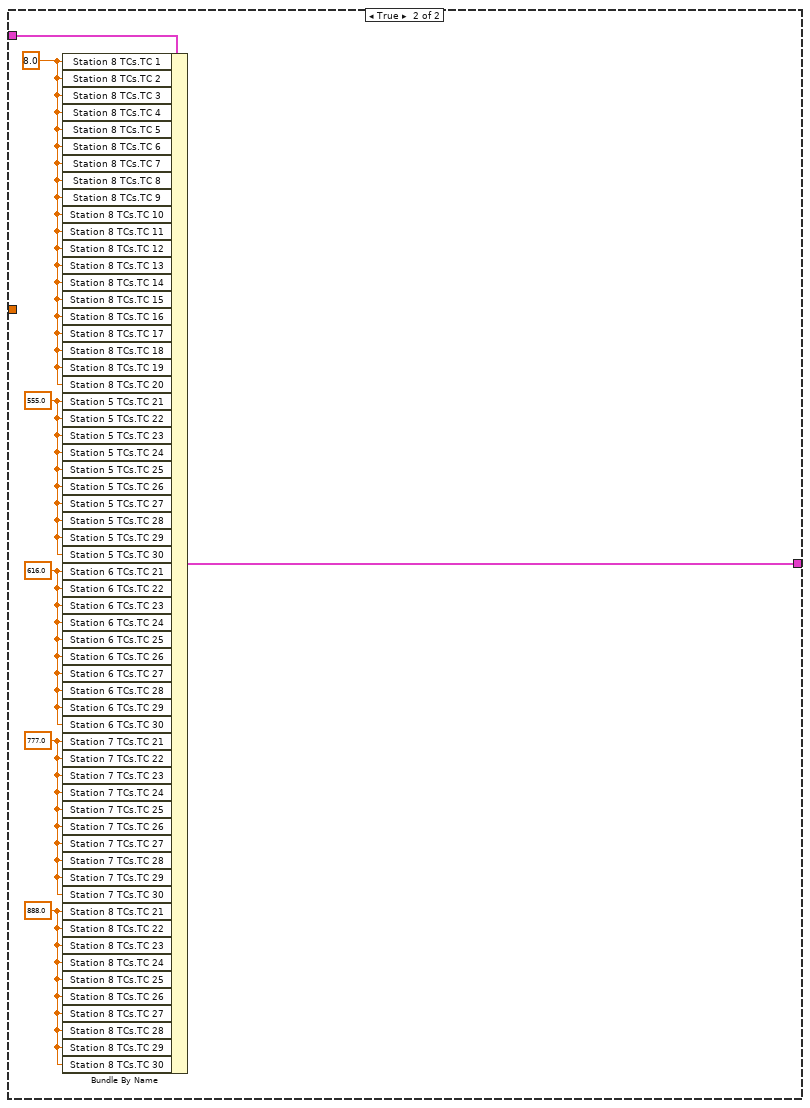
[diagram p2: hidden frame]
diagram:
  n1 = Unbundle By Name("MX") -> ("Base Time"=w8:i32)
  n2 = call "MX100 Filter Data.vi"("Base Time"=w8, "error in (no error)"="Error In", "Measurement Values in"="Measurement Values in", "Measurement Date Times"="Measurement Date Times") -> ("error out"=→"Error Out":errorcluster, "MX100 Data"=w7:T3)  [unwired: 6 in]
  n3 = Bundle By Name(cluster="MX", "MX100 Data"=w7) -> (w3:T2)
  n4 = Unbundle By Name(w3) -> ("MX100 Data.Measurement Values out"=w9:dbl[])
  n5 = case shown="False" "Debug" {
    tunnel: "Chamber 1 Data in in" -> [w135 w142]
    tunnel: [w134 w141] -> w11
    tunnel: w9 -> [w73 _]
    frame False {
      n6 = Index Array(array=w73, index #1=0 ("index"), index #2=1 ("index"), index #3=2 ("index"), index #4=3 ("index"), index #5=4 ("index"), index #6=5 ("index"), index #7=6 ("index"), index #8=7 ("index"), index #9=8 ("index"), index #10=9 ("index"), index #11=10 ("index"), index #12=11 ("index"), index #13=12 ("index"), index #14=13 ("index"), index #15=14 ("index"), index #16=15 ("index"), index #17=16 ("index"), index #18=17 ("index"), index #19=18 ("index"), index #20=19 ("index"), index #21=20 ("index"), index #22=21 ("index"), index #23=22 ("index"), index #24=23 ("index"), index #25=24 ("index"), index #26=25 ("index"), index #27=26 ("index"), index #28=27 ("index"), index #29=28 ("index"), index #30=29 ("index"), index #31=30 ("index"), index #32=31 ("index"), index #33=32 ("index"), index #34=33 ("index"), index #35=34 ("index"), index #36=35 ("index"), index #37=36 ("index"), index #38=37 ("index"), index #39=38 ("index"), index #40=39 ("index"), index #41=40 ("index"), index #42=41 ("index"), index #43=42 ("index"), index #44=43 ("index"), index #45=44 ("index"), index #46=45 ("index"), index #47=46 ("index"), index #48=47 ("index"), index #49=48 ("index"), index #50=49 ("index"), index #51=50 ("index"), index #52=51 ("index"), index #53=52 ("index"), index #54=53 ("index"), index #55=54 ("index"), index #56=55 ("index"), index #57=56 ("index"), index #58=57 ("index"), index #59=58 ("index"), index #60=59 ("index")) -> (element #1=w72:dbl, element #2=w71:dbl, element #3=w70:dbl, element #4=w69:dbl, element #5=w68:dbl, element #6=w67:dbl, element #7=w66:dbl, element #8=w65:dbl, element #9=w64:dbl, element #10=w63:dbl, element #11=w62:dbl, element #12=w61:dbl, element #13=w60:dbl, element #14=w59:dbl, element #15=w58:dbl, element #16=w57:dbl, element #17=w56:dbl, element #18=w55:dbl, element #19=w54:dbl, element #20=w53:dbl, element #21=w52:dbl, element #22=w51:dbl, element #23=w50:dbl, element #24=w49:dbl, element #25=w48:dbl, element #26=w47:dbl, element #27=w46:dbl, element #28=w45:dbl, element #29=w44:dbl, element #30=w43:dbl, element #31=w42:dbl, element #32=w41:dbl, element #33=w40:dbl, element #34=w39:dbl, element #35=w38:dbl, element #36=w37:dbl, element #37=w36:dbl, element #38=w35:dbl, element #39=w34:dbl, element #40=w33:dbl, element #41=w32:dbl, element #42=w31:dbl, element #43=w30:dbl, element #44=w29:dbl, element #45=w28:dbl, element #46=w27:dbl, element #47=w26:dbl, element #48=w25:dbl, element #49=w24:dbl, element #50=w23:dbl, element #51=w22:dbl, element #52=w21:dbl, element #53=w20:dbl, element #54=w19:dbl, element #55=w18:dbl, element #56=w17:dbl, element #57=w16:dbl, element #58=w15:dbl, element #59=w14:dbl, element #60=w13:dbl)
      n7 = Bundle By Name(cluster=w135, "Station 8 TCs.TC 1"=w72, "Station 8 TCs.TC 2"=w71, "Station 8 TCs.TC 3"=w70, "Station 8 TCs.TC 4"=w69, "Station 8 TCs.TC 5"=w68, "Station 8 TCs.TC 6"=w67, "Station 8 TCs.TC 7"=w66, "Station 8 TCs.TC 8"=w65, "Station 8 TCs.TC 9"=w64, "Station 8 TCs.TC 10"=w63, "Station 8 TCs.TC 11"=w62, "Station 8 TCs.TC 12"=w61, "Station 8 TCs.TC 13"=w60, "Station 8 TCs.TC 14"=w59, "Station 8 TCs.TC 15"=w58, "Station 8 TCs.TC 16"=w57, "Station 8 TCs.TC 17"=w56, "Station 8 TCs.TC 18"=w55, "Station 8 TCs.TC 19"=w54, "Station 8 TCs.TC 20"=w53, "Station 5 TCs.TC 21"=w52, "Station 5 TCs.TC 22"=w51, "Station 5 TCs.TC 23"=w50, "Station 5 TCs.TC 24"=w49, "Station 5 TCs.TC 25"=w48, "Station 5 TCs.TC 26"=w47, "Station 5 TCs.TC 27"=w46, "Station 5 TCs.TC 28"=w45, "Station 5 TCs.TC 29"=w44, "Station 5 TCs.TC 30"=w43, "Station 6 TCs.TC 21"=w42, "Station 6 TCs.TC 22"=w41, "Station 6 TCs.TC 23"=w40, "Station 6 TCs.TC 24"=w39, "Station 6 TCs.TC 25"=w38, "Station 6 TCs.TC 26"=w37, "Station 6 TCs.TC 27"=w36, "Station 6 TCs.TC 28"=w35, "Station 6 TCs.TC 29"=w34, "Station 6 TCs.TC 30"=w33, "Station 7 TCs.TC 21"=w32, "Station 7 TCs.TC 22"=w31, "Station 7 TCs.TC 23"=w30, "Station 7 TCs.TC 24"=w29, "Station 7 TCs.TC 25"=w28, "Station 7 TCs.TC 26"=w27, "Station 7 TCs.TC 27"=w26, "Station 7 TCs.TC 28"=w25, "Station 7 TCs.TC 29"=w24, "Station 7 TCs.TC 30"=w23, "Station 8 TCs.TC 21"=w22, "Station 8 TCs.TC 22"=w21, "Station 8 TCs.TC 23"=w20, "Station 8 TCs.TC 24"=w19, "Station 8 TCs.TC 25"=w18, "Station 8 TCs.TC 26"=w17, "Station 8 TCs.TC 27"=w16, "Station 8 TCs.TC 28"=w15, "Station 8 TCs.TC 29"=w14, "Station 8 TCs.TC 30"=w13) -> (w134:T4)
    }
    frame True {
      w136 = 888.0 ("Station 7 TCs.TC 21")
      w137 = 777.0 ("Station 7 TCs.TC 21")
      w138 = 616.0 ("Station 6 TCs.TC 21")
      w139 = 555.0 ("Station 5 TCs.TC 21")
      w140 = 8.0 ("Station 8 TCs.TC 1")
      n8 = Bundle By Name(cluster=w142, "Station 8 TCs.TC 1"=w140, "Station 8 TCs.TC 2"=w140, "Station 8 TCs.TC 3"=w140, "Station 8 TCs.TC 4"=w140, "Station 8 TCs.TC 5"=w140, "Station 8 TCs.TC 6"=w140, "Station 8 TCs.TC 7"=w140, "Station 8 TCs.TC 8"=w140, "Station 8 TCs.TC 9"=w140, "Station 8 TCs.TC 10"=w140, "Station 8 TCs.TC 11"=w140, "Station 8 TCs.TC 12"=w140, "Station 8 TCs.TC 13"=w140, "Station 8 TCs.TC 14"=w140, "Station 8 TCs.TC 15"=w140, "Station 8 TCs.TC 16"=w140, "Station 8 TCs.TC 17"=w140, "Station 8 TCs.TC 18"=w140, "Station 8 TCs.TC 19"=w140, "Station 8 TCs.TC 20"=w140, "Station 5 TCs.TC 21"=w139, "Station 5 TCs.TC 22"=w139, "Station 5 TCs.TC 23"=w139, "Station 5 TCs.TC 24"=w139, "Station 5 TCs.TC 25"=w139, "Station 5 TCs.TC 26"=w139, "Station 5 TCs.TC 27"=w139, "Station 5 TCs.TC 28"=w139, "Station 5 TCs.TC 29"=w139, "Station 5 TCs.TC 30"=w139, "Station 6 TCs.TC 21"=w138, "Station 6 TCs.TC 22"=w138, "Station 6 TCs.TC 23"=w138, "Station 6 TCs.TC 24"=w138, "Station 6 TCs.TC 25"=w138, "Station 6 TCs.TC 26"=w138, "Station 6 TCs.TC 27"=w138, "Station 6 TCs.TC 28"=w138, "Station 6 TCs.TC 29"=w138, "Station 6 TCs.TC 30"=w138, "Station 7 TCs.TC 21"=w137, "Station 7 TCs.TC 22"=w137, "Station 7 TCs.TC 23"=w137, "Station 7 TCs.TC 24"=w137, "Station 7 TCs.TC 25"=w137, "Station 7 TCs.TC 26"=w137, "Station 7 TCs.TC 27"=w137, "Station 7 TCs.TC 28"=w137, "Station 7 TCs.TC 29"=w137, "Station 7 TCs.TC 30"=w137, "Station 8 TCs.TC 21"=w136, "Station 8 TCs.TC 22"=w136, "Station 8 TCs.TC 23"=w136, "Station 8 TCs.TC 24"=w136, "Station 8 TCs.TC 25"=w136, "Station 8 TCs.TC 26"=w136, "Station 8 TCs.TC 27"=w136, "Station 8 TCs.TC 28"=w136, "Station 8 TCs.TC 29"=w136, "Station 8 TCs.TC 30"=w136) -> (w141:T4)
    }
  }
  "Chamber 1 Data out" <- w11
